vi "Read Array Of Tag Elements.vi"(6 "error text in":string, 8 "error in":errorcluster, 10 "tag name":string, 11 "node in":refnum<k20>) -> (0 "error out":errorcluster, 3 "array of elements":refnum<k20>[](array[refnum]))   [LabVIEW 2020, in "ARINC 429 Import.lvlib"]
uses:
  ARINC 429 Import.lvlib
  <resource>/objmgr/DOMUserDefRef.rc
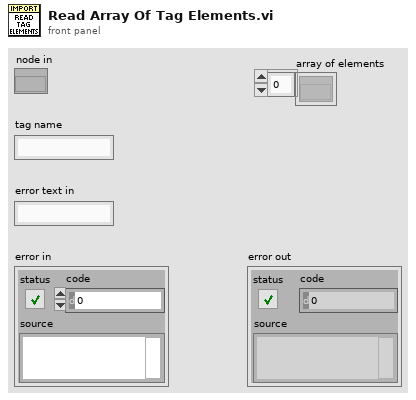
[diagram p1: front panel]
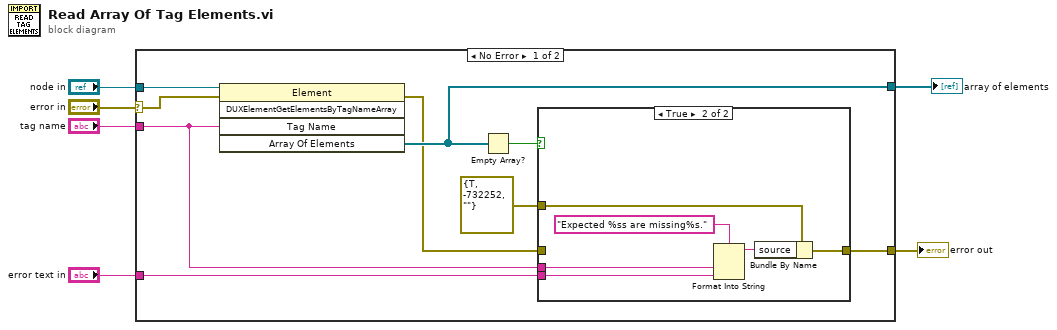
[diagram p0: block diagram]
diagram:
  n1 = case shown="No Error" "error in" {
    selector: "error in" -> [w10 w23]
    tunnel: [w15 w23] -> w5
    tunnel: [w12 _] -> w4
    tunnel: "node in" -> [w11 _]
    tunnel: "tag name" -> [w8 _]
    tunnel: "error text in" -> [w7 _]
    frame No Error {
      n2 = invoke class="Element" method="DUXElementGetElementsByTagNameArray"(reference=w11, error in=w10, "Tag Name"=w8) -> (error out=w9:errorcluster, "Array Of Elements"=w12:refnum<k20>[])  [unwired: 2 in, 3 out]
      n3 = Empty Array?(array=w12) -> (empty?=w13:bool)
      n4 = case shown="True" w13 {
        tunnel: errorcluster {"status"=TRUE, "code"=-732252, "source"=""} ("error constant") -> [_ w21]
        tunnel: [w16 w22] -> w15
        tunnel: w9 -> [w16 _]
        tunnel: w8 -> [_ w19]
        tunnel: w7 -> [_ w17]
        frame False {
        }
        frame True {
          n5 = Format Into String(format string="Expected %ss are missing%s." ("source"), w19, w17) -> (resulting string=w20:string)  [unwired: 2 in, 1 out]
          n6 = Bundle By Name(cluster=w21, "source"=w20) -> (w22:errorcluster)
        }
      }
    }
    frame Error {
    }
  }
  "error out" <- w5
  "array of elements" <- w4
